vi "ASK_XSRPLoopback.vi"(5 "xsrpip":string, 7 "pcip":string, 8 "error in (no error)":errorcluster caption="错误输入（无错误）", 10 "tx_data":cdb[](array[numeric]) format="%#_13g", 11 "PathIn":path) -> (0 "error out":errorcluster caption="错误输出", 1 "ERR_CODE":dbl, 2 "rxdataIQ":cdb[](array[numeric]), 3 "PathOut":path)   [LabVIEW 2015]
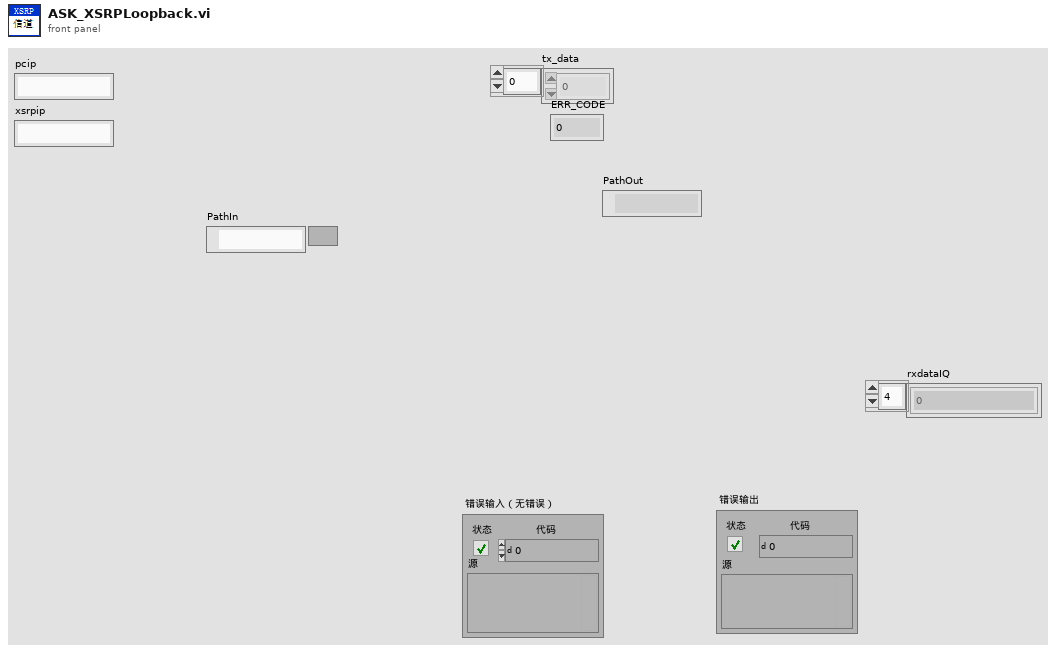
[diagram p1: front panel]
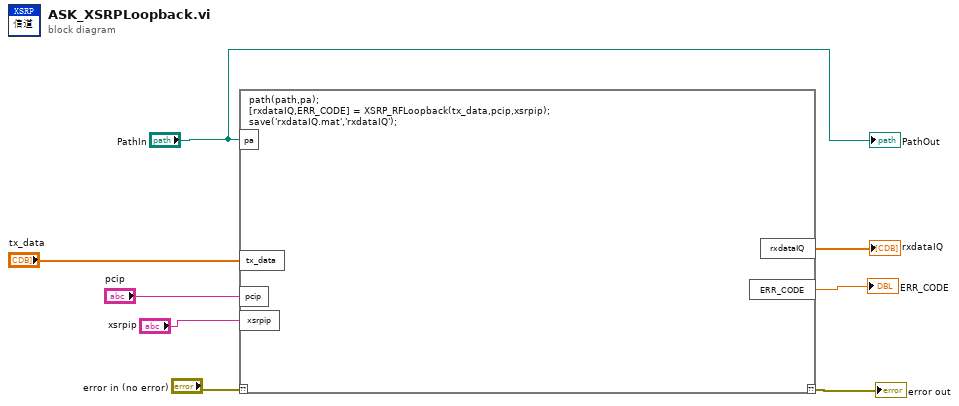
[diagram p0: block diagram]
diagram:
  n1 = script code="path(path,pa);\n[rxdataIQ,ERR_CODE] = XSRP_RFLoopback(tx_data,pcip,xsrpip);\nsave('rxdataIQ.mat','rxdataIQ');"("??"="error in (no error)", "pa"="PathIn", "tx_data"="tx_data", "pcip"="pcip", "xsrpip"="xsrpip") -> ("??"=→"error out":errorcluster, "rxdataIQ"=→"rxdataIQ":cdb[], "ERR_CODE"=→"ERR_CODE":dbl)
  "PathOut" <- "PathIn"
